vi "图片浏览器1.vi"() -> ()   [LabVIEW 2018]
panel:
  in  "后一张":bool
  in  "前一张":bool
  in  "打开":bool
  out "select your shoes":picture
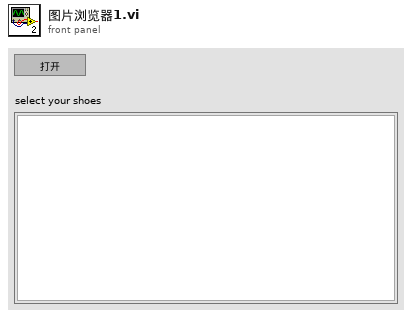
[diagram p1: front panel]
types:
  T1 = typedef "imagedata.ctl" = cluster{"image type":i32, "image depth":i32, "image":u8[], "mask":u8[], "colors":u32[], "Rectangle":cluster{"left":i16, "top":i16, "right":i16, "bottom":i16}}
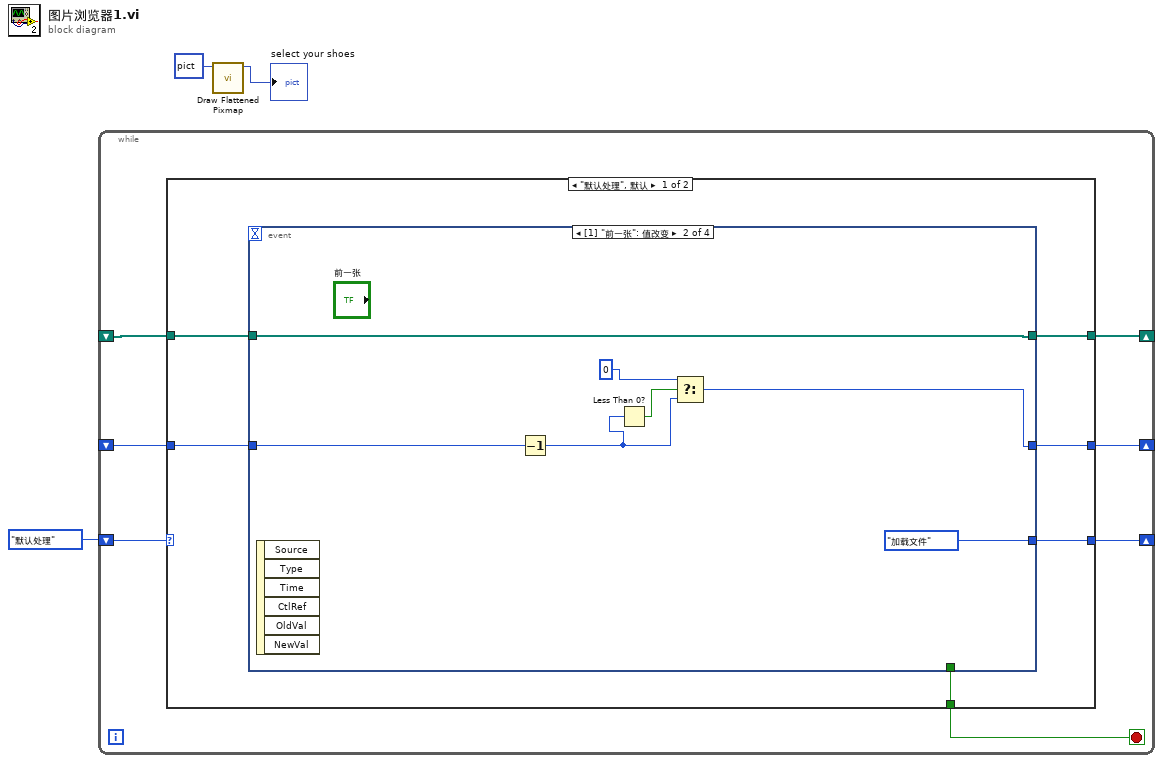
[diagram p0: block diagram]
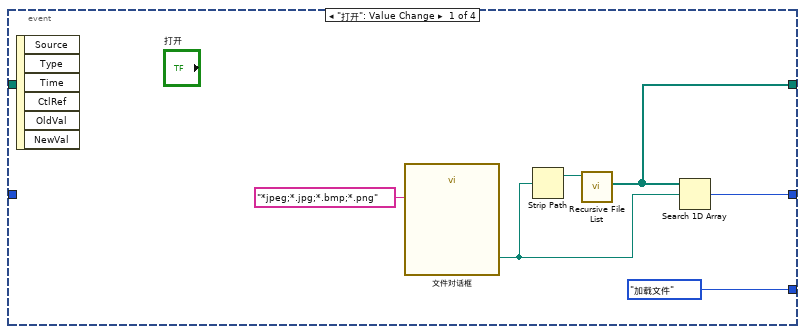
[diagram p2: hidden frame]
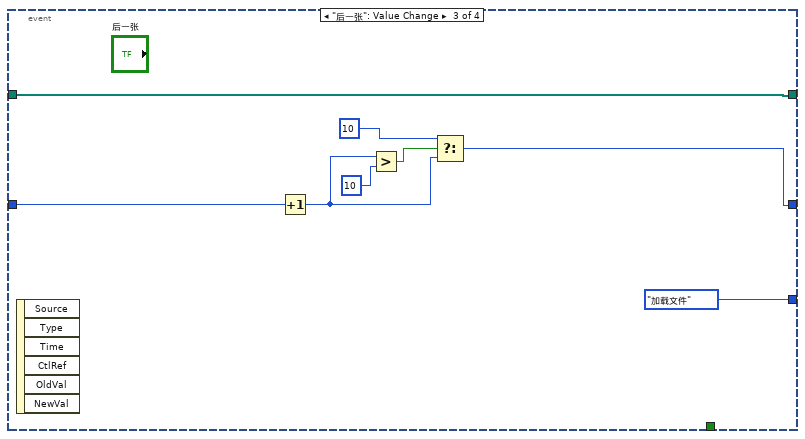
[diagram p3: hidden frame]
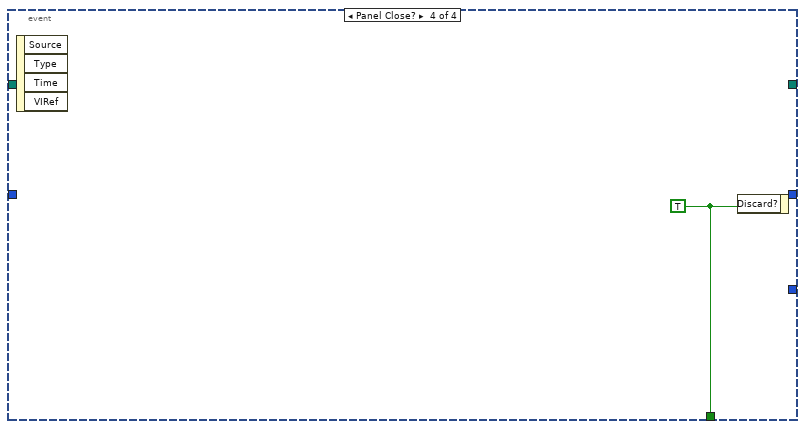
[diagram p4: hidden frame]
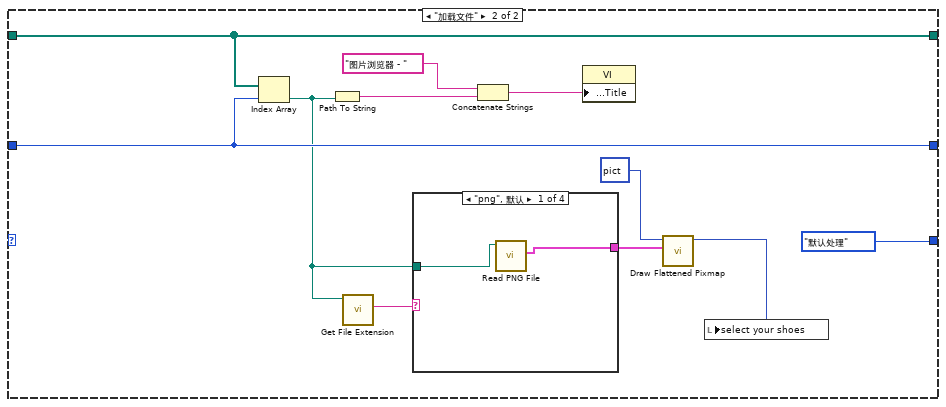
[diagram p5: hidden frame]
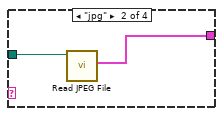
[diagram p6: hidden frame]
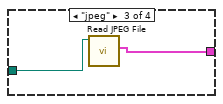
[diagram p7: hidden frame]
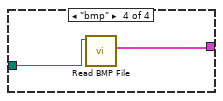
[diagram p8: hidden frame]
diagram:
  n1 = while {
    shift-right: [w10] -> _
    shift-left: _ -> [w8]
    shift-right: [w9] -> _
    shift-left: _ -> [w7]
    shift-right: [w6] -> _
    shift-left: enum16{"默认处理", "加载文件"}."默认处理" -> [w5]
    stop <- w4 stop-if-true
    n2 = case shown="\"默认处理\", 默认" w5 {
      tunnel: [w16 w45] -> w10
      tunnel: [w15 w44] -> w9
      tunnel: w8 -> [w14 w45]
      tunnel: w7 -> [w13 w44]
      tunnel: [w12 enum16{"默认处理", "加载文件"}."默认处理"] -> w6
      tunnel: [w11 _] -> w4
      frame "默认处理", Default {
        n3 = event shown="[1] \"前一张\": 值改变" {
          selector: _ -> [_ _ _ _]
          dyn-events: _ -> [_ _ _ _]
          timeout: _ -> [_ _ _ _]
          tunnel: [w19 w29 w37 _] -> w16
          tunnel: [w18 w24 w34 _] -> w15
          tunnel: w14 -> [_ w29 w37 _]
          tunnel: w13 -> [_ w28 w36 _]
          tunnel: [enum16{"默认处理", "加载文件"}."加载文件" enum16{"默认处理", "加载文件"}."加载文件" enum16{"默认处理", "加载文件"}."加载文件" _] -> w12
          tunnel: [_ _ _ w38] -> w11
          event "打开": Value Change {
            n4 = event-data() -> ()  [unwired: 1 in, 6 out]
            n5 = call "文件对话框"("pattern (all files)"="*jpeg;*.jpg;*.bmp;*.png") -> ("selected path"=w20:path)  [unwired: 11 in, 3 out]
            n6 = Strip Path(path=w20) -> (stripped path=w21:path)  [unwired: 1 out]
            n7 = call <vilib>:"Recursive File List.vi"("Folder Path"=w21) -> ("All Files in Dir"=w19:path[])  [unwired: 6 in, 4 out]
            n8 = Search 1D Array(1D array=w19, element=w20) -> (index of element=w18:i32)  [unwired: 1 in]
          }
          event "前一张": Value Change {
            n9 = event-data() -> ()  [unwired: 1 in, 6 out]
            n10 = Decrement(x=w28) -> (x-1=w26:i32)
            n11 = Less Than 0?(x=w26) -> (x < 0?=w27:bool)
            n12 = Select(t=0, s=w27, f=w26) -> (s? t:f=w24:i32)
          }
          event "后一张": Value Change {
            n13 = event-data() -> ()  [unwired: 1 in, 6 out]
            n14 = Increment(x=w36) -> (x+1=w31:i32)
            n15 = Greater?(x=w31, y=10) -> (0:w30:bool)
            n16 = Select(t=10, s=w30, f=w31) -> (s? t:f=w34:i32)
          }
          event Panel Close? {
            w38 = TRUE
            n17 = event-data() -> ()  [unwired: 1 in, 4 out]
            n18 = event-data("Discard?"=w38) -> ()  [unwired: 1 in, 1 out]
          }
        }
      }
      frame "加载文件" {
        n19 = Index Array(array=w45, index=w44) -> (element=w43:path)
        n20 = Path To String(path=w43) -> (string=w47:string)
        n21 = call <vilib>:"Get File Extension.vi"("file"=w43) -> ("lowercase file extension"=w41:string)  [unwired: 6 in, 4 out]
        n22 = case shown="\"png\", 默认" w41 {
          tunnel: w43 -> [w50 w53 w54 w56]
          tunnel: [w51 w52 w55 w57] -> w42
          frame "png", Default {
            n23 = call <vilib>:"Read PNG File.vi"("path to PNG file"=w50) -> ("image data"=w51:T1)  [unwired: 8 in, 2 out]
          }
          frame "jpg" {
            n24 = call <vilib>:"Read JPEG File.vi"("path to JPEG file"=w53) -> ("image data"=w52:T1)  [unwired: 8 in, 2 out]
          }
          frame "jpeg" {
            n25 = call <vilib>:"Read JPEG File.vi"("path to JPEG file"=w54) -> ("image data"=w55:T1)  [unwired: 8 in, 2 out]
          }
          frame "bmp" {
            n26 = call <vilib>:"Read BMP File.vi"("path to BMP file"=w56) -> ("image data"=w57:T1)  [unwired: 8 in, 2 out]
          }
        }
        n27 = Concatenate Strings("图片浏览器 - " ("字符串"), w47) -> (w39:string)
        n28 = property class="VI"("Front Panel.Title"=w39) -> ()  [unwired: 2 in, 2 out]
        n29 = call <vilib>:"Draw Flattened Pixmap.vi"("image data"=w42, "picture"=picture data[5B]) -> ("new picture"=w48:picture)  [unwired: 7 in]
        n30 = local write "select your shoes"(w48) -> ()
      }
    }
  }
  n31 = call <vilib>:"Draw Flattened Pixmap.vi"("picture"=picture data[5B]) -> ("new picture"=→"select your shoes":picture)  [unwired: 8 in]
